vi "PID Straight.vi"(6 "Reinitialize":bool, 7 "Target Angle":dbl, 8 "Error In":errorcluster, 9 "Gyro Angle":dbl, 10 "Current Distance":dbl, 11 "Target Distance":dbl) -> (0 "Error Out":errorcluster, 2 "Right Power":dbl, 3 "Left Power":dbl)   [LabVIEW 2016]
uses:
  <vilib>/addons/control/pid/pid.llb/PID (DBL).vi
  <vilib>/addons/control/pid/NI_PID_pid.lvlib
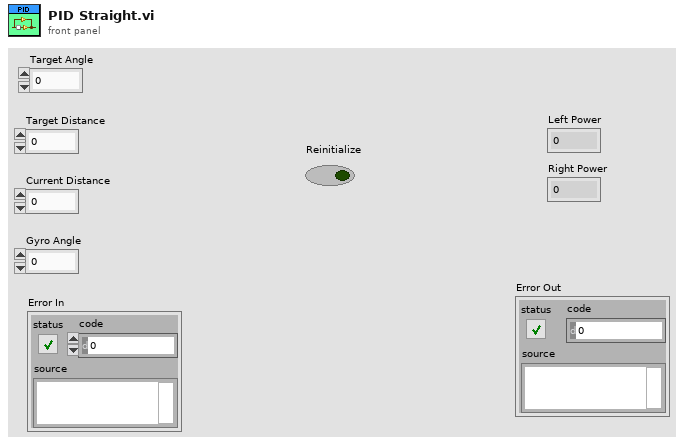
[diagram p1: front panel]
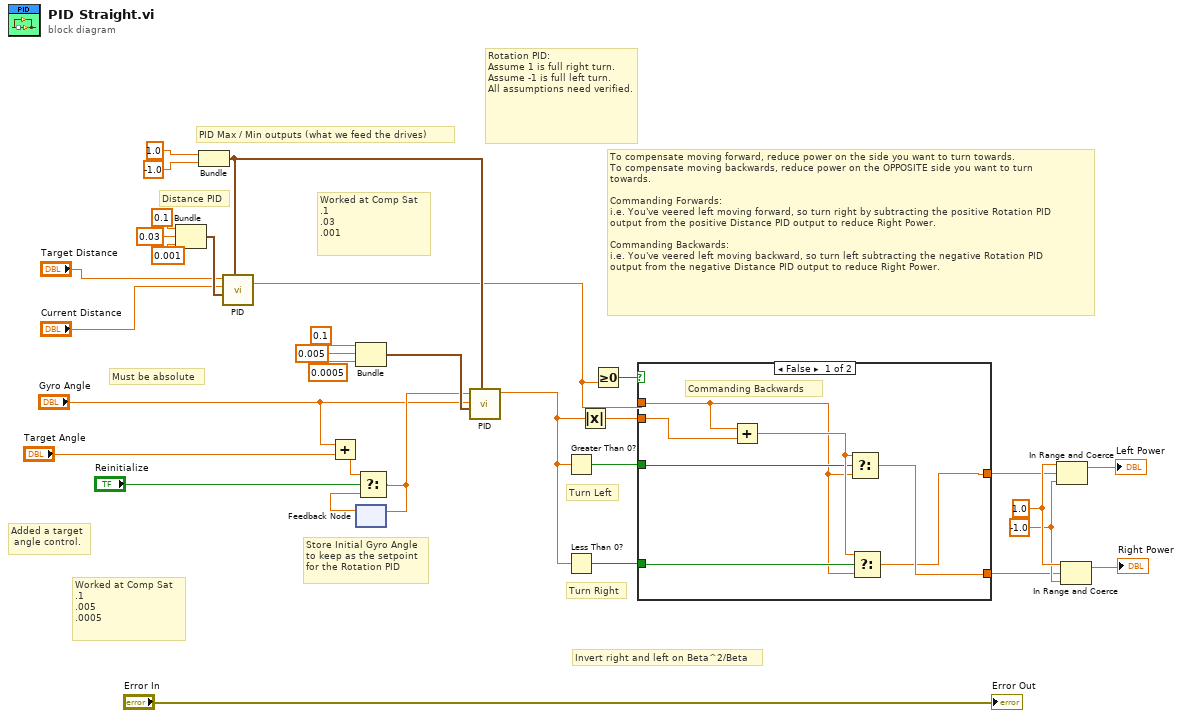
[diagram p0: block diagram]
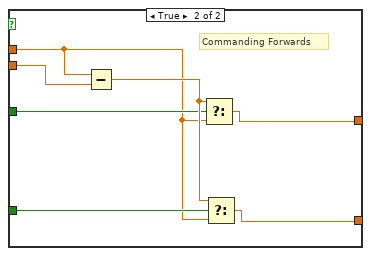
[diagram p2: hidden frame]
diagram:
  w15 = -1.0
  w16 = 1.0
  # "Added a target\n angle control."
  # "Worked at Comp Sat\n.1\n.03\n.001"
  # "Worked at Comp Sat\n.1\n.005\n.0005"
  # "Invert right and left on Beta^2/Beta"
  # "Turn Right"
  # "Turn Left"
  # "To compensate moving forward, reduce power on the side you want to turn towards.\nTo compensate moving backwards, reduce power on the OPPOSITE side you want to turn\ntowards.\n\nCommanding Forwards:\ni.e. You've veered left moving forward, so turn right by subtracting the positive Rotation PID\noutput from the positive Distance PID output to reduce Right Power.\n\nCommanding Backwards:\ni.e. You've veered left moving backward, so turn left subtracting the negative Rotation PID \noutput from the negative Distance PID output to reduce Right Power."
  # "PID Max / Min outputs (what we feed the drives)"
  # "Must be absolute"
  # "Rotation PID:\nAssume 1 is full right turn.\nAssume -1 is full left turn.\nAll assumptions need verified."
  # "Distance PID"
  # "Store Initial Gyro Angle\nto keep as the setpoint\nfor the Rotation PID"
  n1 = Bundle(0.1, 0.03, 0.001) -> (w27:cluster{dbl, dbl, dbl})  [unwired: 1 in]
  n2 = Bundle(1.0, -1.0) -> (w20:cluster{dbl, dbl})  [unwired: 1 in]
  n3 = call-poly <vilib>:"PID.vi"("output range"=w20, "PID gains"=w27, "process variable"="Current Distance", "setpoint"="Target Distance") -> ("output"=w14:dbl)  [unwired: 6 in, 1 out]
  n4 = Add(x="Gyro Angle", y="Target Angle") -> (x+y=w1:dbl)
  n5 = Bundle(0.1, 0.005, 0.0005) -> (w21:cluster{dbl, dbl, dbl})  [unwired: 1 in]
  n6 = feedback #1() -> (w6:dbl)  [unwired: 1 in]
  n7 = Select(t=w1, s="Reinitialize", f=w6) -> (s? t:f=w4:dbl)
  n8 = feedback-in #1(w4) -> ()
  n9 = call-poly <vilib>:"PID.vi"("output range"=w20, "PID gains"=w21, "process variable"="Gyro Angle", "setpoint"=w4) -> ("output"=w8:dbl)  [unwired: 6 in, 1 out]
  n10 = Greater Than 0?(x=w8) -> (x > 0?=w10:bool)
  n11 = Less Than 0?(x=w8) -> (x < 0?=w9:bool)
  n12 = Absolute Value(x=w8) -> (abs(x)=w13:dbl)
  n13 = Greater Or Equal To 0?(x=w14) -> (x >= 0?=w19:bool)
  n14 = case shown="False" w19 {
    tunnel: w13 -> [w36 w46]
    tunnel: w14 -> [w33 w40]
    tunnel: [w35 w44] -> w12
    tunnel: [w34 w43] -> w11
    tunnel: w10 -> [w38 w42]
    tunnel: w9 -> [w37 w41]
    frame False {
      # "Commanding Backwards"
      n15 = Add(x=w33, y=w36) -> (x+y=w39:dbl)
      n16 = Select(t=w39, s=w38, f=w33) -> (s? t:f=w35:dbl)
      n17 = Select(t=w39, s=w37, f=w33) -> (s? t:f=w34:dbl)
    }
    frame True {
      # "Commanding Forwards"
      n18 = Subtract(x=w40, y=w46) -> (x-y=w45:dbl)
      n19 = Select(t=w45, s=w42, f=w40) -> (s? t:f=w43:dbl)
      n20 = Select(t=w45, s=w41, f=w40) -> (s? t:f=w44:dbl)
    }
  }
  n21 = In Range and Coerce(upper limit=w16, x=w11, lower limit=w15) -> (coerced(x)=→"Left Power":dbl)  [unwired: 1 out]
  n22 = In Range and Coerce(upper limit=w16, x=w12, lower limit=w15) -> (coerced(x)=→"Right Power":dbl)  [unwired: 1 out]
  "Error Out" <- "Error In"
